vi "GCMPlugin_GetPluginName.vi"(8 "error in (no error)":errorcluster, 11 "TemplatePlugin in":refnum<class "VIWindowProperties.lvclass">) -> (0 "error out":errorcluster, 2 "PluginName":string, 3 "TemplatePlugin out":refnum<class "VIWindowProperties.lvclass">)   [LabVIEW 2014, in "VIWindowProperties.lvlib" / "VIWindowProperties.lvclass"]
uses:
  VIWindowProperties.lvclass
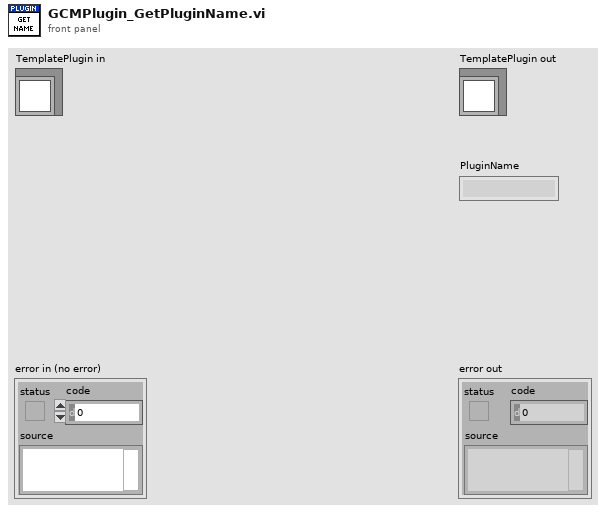
[diagram p1: front panel]
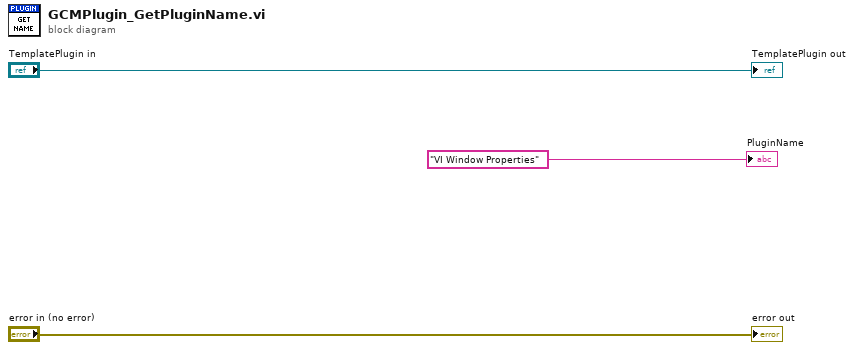
[diagram p0: block diagram]
diagram:
  "error out" <- "error in (no error)"
  "TemplatePlugin out" <- "TemplatePlugin in"
  "PluginName" <- "VI Window Properties"
